vi "Global Variables.vi"() -> ()   [LabVIEW 2014]
doc: "This global VI can contain as many global variables as you need. Place a control on the panel, give it a good name. To read or write to it from a VI, drag the icon to the diagram of that VI. You can also drag from the project. Click on the node to change which global you access. You shouldn't have multiple locations writing to a global or it will cause a race-condition."
uses:
  <vilib>/Rock Robotics/WPI/DriverStation/WPI_DriverStationRobotMode2.ctl
panel:
  out "Driver Start":bool
  out "Heading to Maintain":dbl
  out "NavX Yaw":dbl
  out "Driver Joystick X2":dbl
  out "Driver Joystick Y1":dbl
  out "Driver Joystick X1":dbl
  out "Rot BR":dbl
  out "Drive BR":dbl
  out "Rot BL":dbl
  out "Drive BL":dbl
  out "Rot FR":dbl
  out "Drive FR":dbl
  out "Rot FL":dbl
  out "Drive FL":dbl
  in  "Robot Mode":T1
  # "Sensors"
  # "Misc"
  # "Drive Motors"
  # "Driver Controller"
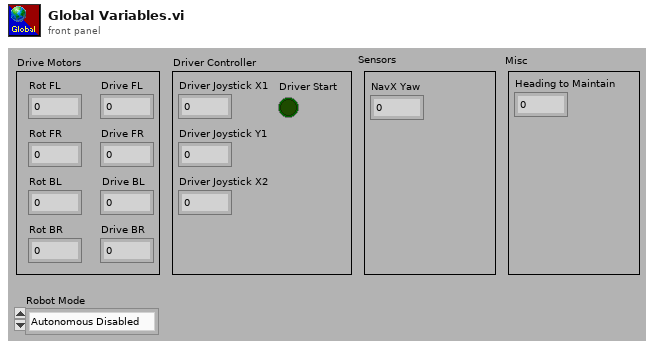
[diagram p1: front panel]
types:
  T1 = typedef "WPI_DriverStationRobotMode2.ctl" = enum16{"Autonomous Disabled", "Autonomous Enabled", "Teleop Disabled", "Teleop Enabled", "Disconnected", "Finish", "Test Disabled", "Test Enabled", "Emergency Stopped"}
diagram:
